vi "Get Menu Item VI.vi"(7 "Menu Item":string, 8 "error in (no error)":errorcluster, 9 "GUID":string, 10 "Item Ref":T1 format="%.0x", 11 "System Explorer Dispatcher Implementation in":refnum<class "System Explorer Dispatcher.lvclass">) -> (0 "error out":errorcluster, 2 "menu item reference":refnum<vi>, 3 "System Explorer Dispatcher Implementation out":refnum<class "System Explorer Dispatcher.lvclass">)   [LabVIEW 2020, in "AIM ARINC 664 System Explorer.lvlib" / "Implementation.lvlib" / "System Explorer Dispatcher.lvclass"]
uses:
  System Explorer Dispatcher.lvclass
  <vilib>/NI VeriStand/Custom Device API/Custom Device Item Ref.ctl
  Scripting/Constants.vi
  System Explorer/RTM/Import Configuration RTM.vi
  System Explorer/RTM/Configure Payload Frames RTM.vi
  System Explorer/RTM/Add RxUDP Information RTM.vi
  Scripting/AIM ARINC 664 Scripting.lvlib
  Implementation.lvlib
  <vilib>/NI VeriStand/Custom Device API/Custom Device API.lvlib
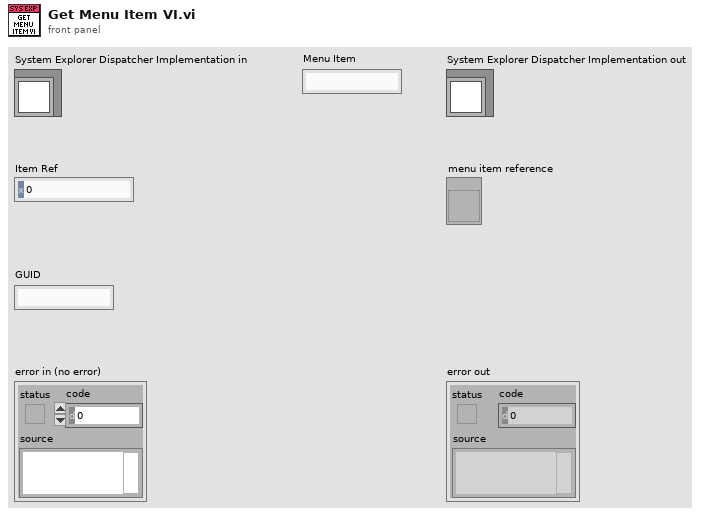
[diagram p1: front panel]
types:
  T1 = typedef "Custom Device API.lvlib/Custom Device Item Ref.ctl" = u64
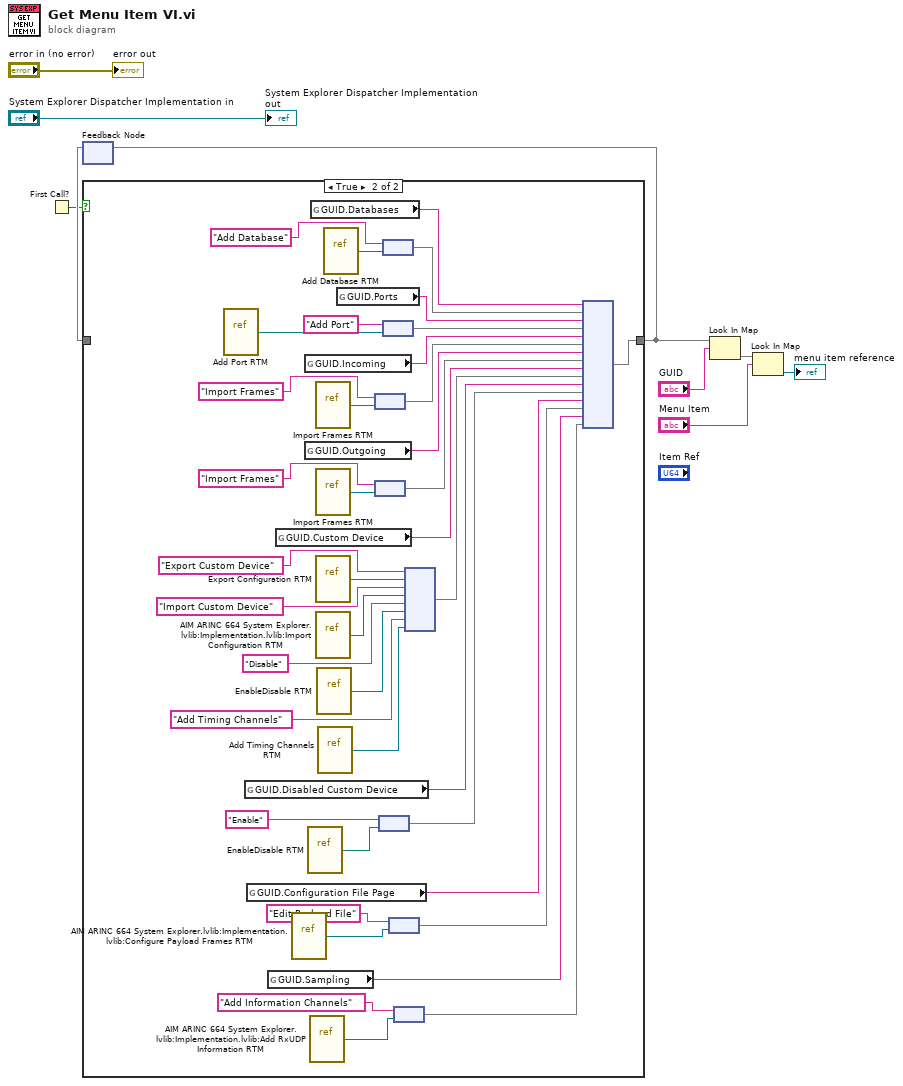
[diagram p0: block diagram]
diagram:
  n1 = First Call?() -> (First Call?: T/F=w1:bool)
  n2 = feedback #1() -> (w7:map{string, map{string, refnum<vi>}})  [unwired: 1 in]
  n3 = case shown="True" w1 {
    tunnel: [w10 w49] -> w8
    tunnel: w7 -> [w10 _]
    frame False {
    }
    frame True {
      n4 = vi-ref "Add Port RTM.vi"() -> (w41:refnum<vi>)
      n5 = global read "Constants.vi" "GUID.Disabled Custom Device"() -> (w23:string)
      n6 = global read "Constants.vi" "GUID.Configuration File Page"() -> (w16:string)
      n7 = global read "Constants.vi" "GUID.Sampling"() -> (w12:string)
      n8 = global read "Constants.vi" "GUID.Custom Device"() -> (w30:string)
      n9 = vi-ref "AIM ARINC 664 System Explorer.lvlib:Implementation.lvlib:Configure Payload Frames RTM.vi"() -> (w18:refnum<vi>)
      n10 = global read "Constants.vi" "GUID.Incoming"() -> (w38:string)
      n11 = global read "Constants.vi" "GUID.Outgoing"() -> (w34:string)
      n12 = vi-ref "EnableDisable RTM.vi"() -> (w25:refnum<vi>)
      n13 = vi-ref "AIM ARINC 664 System Explorer.lvlib:Implementation.lvlib:Add RxUDP Information RTM.vi"() -> (w13:refnum<vi>)
      n14 = global read "Constants.vi" "GUID.Databases"() -> (w48:string)
      n15 = vi-ref "Import Frames RTM.vi"() -> (w40:refnum<vi>)
      n16 = vi-ref "Import Frames RTM.vi"() -> (w35:refnum<vi>)
      n17 = vi-ref "Export Configuration RTM.vi"() -> (w32:refnum<vi>)
      n18 = vi-ref "AIM ARINC 664 System Explorer.lvlib:Implementation.lvlib:Import Configuration RTM.vi"() -> (w28:refnum<vi>)
      n19 = vi-ref "EnableDisable RTM.vi"() -> (w26:refnum<vi>)
      n20 = vi-ref "Add Timing Channels RTM.vi"() -> (w20:refnum<vi>)
      n21 = vi-ref "Add Database RTM.vi"() -> (w44:refnum<vi>)
      n22 = global read "Constants.vi" "GUID.Ports"() -> (w47:string)
      n23 = node("Import Frames", w40) -> (w37:map{string, refnum<vi>})
      n24 = node("Import Frames", w35) -> (w33:map{string, refnum<vi>})
      n25 = node("Enable", w25) -> (w22:map{string, refnum<vi>})
      n26 = node("Add Database", w44) -> (w46:map{string, refnum<vi>})
      n27 = node("Add Port", w41) -> (w42:map{string, refnum<vi>})
      n28 = node("Edit Payload File" ("key"), w18) -> (w15:map{string, refnum<vi>})
      n29 = node("Add Information Channels" ("key"), w13) -> (w11:map{string, refnum<vi>})
      n30 = node("Export Custom Device", w32, "Import Custom Device", w28, "Disable", w26, "Add Timing Channels", w20) -> (w19:map{string, refnum<vi>})
      n31 = node(w48, w46, w47, w42, w38, w37, w34, w33, w30, w19, w23, w22, w16, w15, w12, w11) -> (w49:map{string, map{string, refnum<vi>}})
    }
  }
  n32 = feedback-in #1(w8) -> ()
  n33 = Look In Map(map=w8, key="GUID") -> (value=w5:map{string, refnum<vi>})  [unwired: 1 in, 1 out]
  n34 = Look In Map(map=w5, key="Menu Item") -> (value=→"menu item reference":refnum<vi>)  [unwired: 1 in, 1 out]
  "error out" <- "error in (no error)"
  "System Explorer Dispatcher Implementation out" <- "System Explorer Dispatcher Implementation in"
